vi "All Channels.vi"(8 "error in (no error)":errorcluster, 11 "StringGroup in":refnum<class "StringGroup.lvclass">) -> (0 "error out":errorcluster, 2 "All Channels":refnum<class "StringChannel.lvclass">[](array[class]), 3 "StringGroup out":refnum<class "StringGroup.lvclass">)   [LabVIEW 2020, in "Vecto.lvlib" / "StringGroup.lvclass"]
uses:
  StringGroup.lvclass
  StringGroup.lvclass/StringGroup.ctl
  GroupAbstract/GroupAbstract.lvclass
  StringChannel/StringChannel.lvclass
  C:/dev/lv20CE/relink/lv-vecto/Vecto/GroupAbstract/GroupAbstract.lvclass
  C:/dev/lv20CE/relink/lv-vecto/Vecto/StringGroup/StringGroup.lvclass
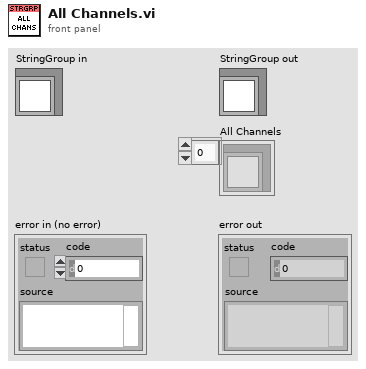
[diagram p1: front panel]
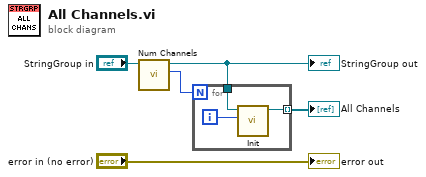
[diagram p0: block diagram]
diagram:
  n1 = call "Num Channels.vi"("GroupAbstract in"="StringGroup in") -> ("Num Channels"=w4:i32, "GroupAbstract out"=w2:refnum<class "StringGroup.lvclass">)  [unwired: 8 in, 1 out]
  "StringGroup out" <- w2
  n2 = for {
    N: w4 -> [_]
    tunnel: w2 -> [w7]
    tunnel: [w6] -> w1 mode=indexing
    i -> [w8]
    n3 = call "Init.vi"("Index"=w8, "Group"=w7) -> ("StringChannel out"=w6:refnum<class "StringChannel.lvclass">)  [unwired: 8 in, 1 out]
  }
  "All Channels" <- w1
  "error out" <- "error in (no error)"
